vi "V_Rail_v2.vi"(8 "Error In":errorcluster, 11 "Read Task":string) -> (0 "Error Out":errorcluster, 3 "DC values":dbl[](array[numeric]) format="%.4p")   [LabVIEW 2021]
uses:
  <vilib>/DAQmx/read.llb/DAQmx Read (Analog 1D Wfm NChan NSamp).vi
  <vilib>/DAQmx/miscellaneous.llb/DAQmx Fill In Error Info.vi
  <vilib>/measure/madcrms.llb/Basic Averaged DC-RMS for N Chan.vi
  <vilib>/measure/NI_MAPro.lvlib
panel:
  out "Output Signal":waveform(dbl)[](graph)=[{"t0"=timestamp(0 s since 1904-01-01), "dt"=0.001, "Y"=[]}]
  # "+15V"
  # "+5V"
  # "+5V_Ref"
  # "+15V_A"
  # "-15V_A"
  # "+17V_A"
  # "-17V_A"
  # "+5V_A"
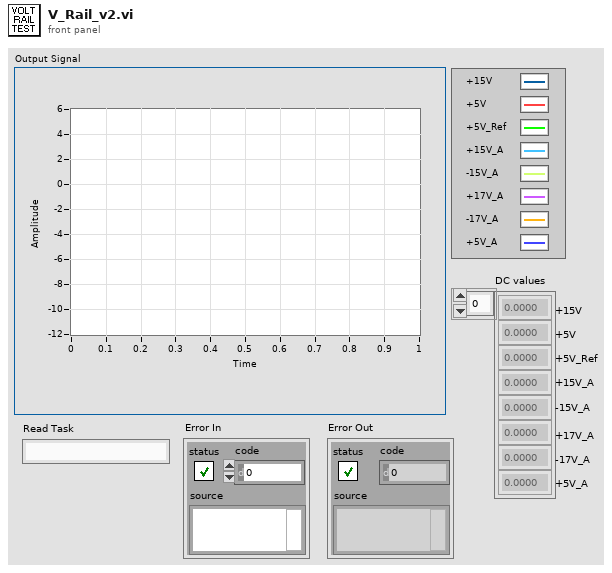
[diagram p1: front panel]
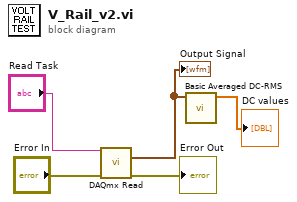
[diagram p0: block diagram]
diagram:
  n1 = call-poly <vilib>:"DAQmx Read.vi"("task/channels in"="Read Task", "error in"="Error In") -> ("data"=w5:waveform(dbl)[], "error out"=→"Error Out":errorcluster)  [unwired: 11 in, 1 out]
  "Output Signal" <- w5
  n2 = call-poly <vilib>:"Basic Averaged DC-RMS.vi"("signals in"=w5) -> ("DC values"=→"DC values":dbl[])  [unwired: 7 in, 3 out]
